vi "Mask XY Graph_Check Boundary.vi"(11 "Boundary":cluster{"X":dbl[], "Y":dbl[]}) -> (2 "Open Boundary":cluster{"X":dbl[], "Y":dbl[]}, 3 "Closed Boundary":cluster{"X":dbl[], "Y":dbl[]})   [LabVIEW 2023]
doc: "Generate Closed Boundary and Open Boundary clusters that can be displayed in an XY Graph."
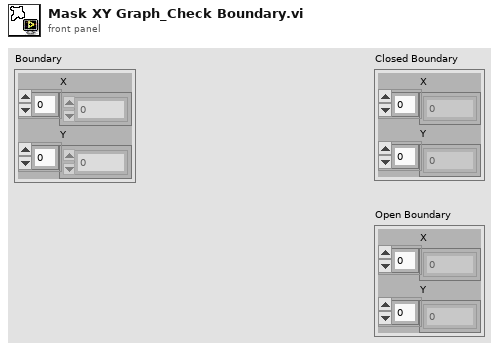
[diagram p1: front panel]
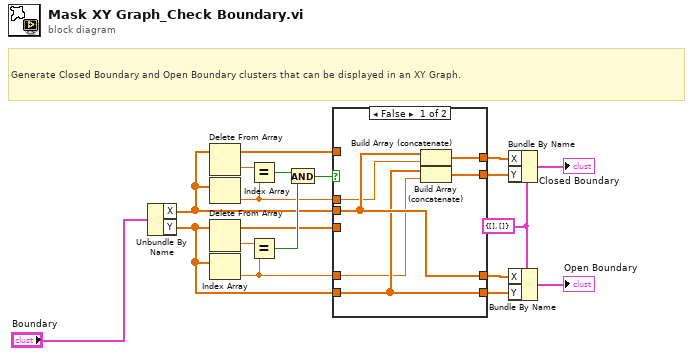
[diagram p0: block diagram]
diagram:
  w1 = cluster{"X":dbl[], "Y":dbl[]} {"X"=[], "Y"=[]} ("Boundary")
  # "Generate Closed Boundary and Open Boundary clusters that can be displayed in an XY Graph."
  n1 = Unbundle By Name("Boundary") -> ("X"=w12:dbl[], "Y"=w9:dbl[])
  n2 = Delete From Array(array=w12) -> (deleted portion=w19:dbl, array with subset deleted=w13:dbl[])  [unwired: 2 in]
  n3 = Index Array(array=w12) -> (element=w11:dbl)  [unwired: 1 in]
  n4 = Delete From Array(array=w9) -> (deleted portion=w18:dbl, array with subset deleted=w5:dbl[])  [unwired: 2 in]
  n5 = Index Array(array=w9) -> (element=w10:dbl)  [unwired: 1 in]
  n6 = Equal?(x=w19, y=w11) -> (x = y?=w17:bool)
  n7 = Equal?(x=w18, y=w10) -> (x = y?=w16:bool)
  n8 = And(x=w17, y=w16) -> (x .and. y?=w14:bool)
  n9 = case shown="False" w14 {
    tunnel: w13 -> [_ w29]
    tunnel: w12 -> [w25 w27]
    tunnel: w11 -> [w24 _]
    tunnel: w10 -> [w20 _]
    tunnel: w9 -> [w21 w26]
    tunnel: [w25 w29] -> w6
    tunnel: w5 -> [_ w28]
    tunnel: [w21 w28] -> w4
    tunnel: [w23 w27] -> w3
    tunnel: [w22 w26] -> w2
    frame False {
      n10 = Build Array (concatenate)(w25, w24) -> (w23:dbl[])
      n11 = Build Array (concatenate)(w21, w20) -> (w22:dbl[])
    }
    frame True {
    }
  }
  n12 = Bundle By Name(cluster=w1, "X"=w3, "Y"=w2) -> (→"Closed Boundary":cluster{"X":dbl[], "Y":dbl[]})
  n13 = Bundle By Name(cluster=w1, "X"=w6, "Y"=w4) -> (→"Open Boundary":cluster{"X":dbl[], "Y":dbl[]})
